vi "WPI_MotorControlOpen NidecBrushless.vi"(6 "Invert":bool, 8 "error in (no error)":errorcluster, 9 "DIO Channel":T1, 10 "PWM Channel":T4) -> (0 "error out":errorcluster, 3 "MotorControlDeviceRef":T2={"DeviceStatus"={"status"=FALSE, "code"=0, "source"=""}, "Type"=enum."PWM", "PWM"={"PWM Channel"=enum."Invalid", "DeadBand"={"Name"="", "maxPositivePwm"=0, "minPositivePwm"=0, "centerPwm"=0, "maxNegativePwm"=0, "minNegativePwm"=0, "angularRange"=0}}, "CAN"={"Device Number"=0, "SetOutput VI Ref"=variant(refnum<vi> refnum), "GetOutput VI Ref"=variant(refnum<vi> refnum), "Enable VI Ref"=variant(refnum<vi> refnum), "Disable VI Ref"=variant(refnum<vi> refnum), "Data"=variant}, "Invert"=FALSE, "DIO PWM"={"PWM \"Enable\" Channel"=enum."Invalid", "DIOChannel"=enum."Invalid", "PWM Rate"=0.0}})   [LabVIEW 2017]
doc: "Creates a reference to the Nidec Brushless motor controller you specify. You must open a reference before using any other VIs on this palette. After you open a reference to the motor controller, you can use the SetOutput and GetOutput VIs to set and get the output voltage of the motor controller, respectively.\n\nThis software is licensed. Open the labview\\readme\\WPI Robotics Library Open Source License.txt file for more information."
uses:
  <vilib>/Rock Robotics/SystemInterfaces/DIO/FPGA_DIOPWMChannel.ctl
  <vilib>/Rock Robotics/WPI/MotorControl/WPI_MotorControlDeviceRef.ctl
  <vilib>/Rock Robotics/WPI/MotorControl/WPI_MotorControlType.ctl
  <vilib>/Rock Robotics/WPI/PWM/WPI_PWMDeadband.ctl
  <vilib>/Rock Robotics/SystemInterfaces/DIO/FPGA_DIOChannel.ctl
  <vilib>/Rock Robotics/SystemInterfaces/NetworkCommunication/NetComm_UsageReport_ResourceType.ctl
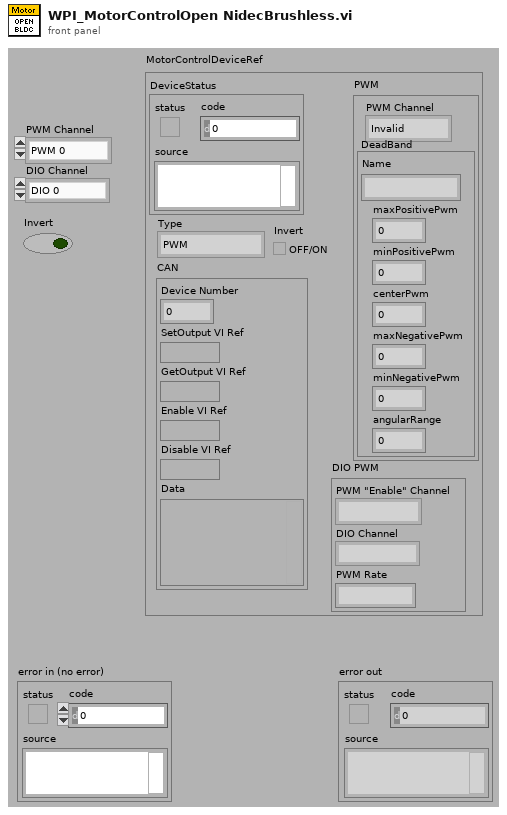
[diagram p1: front panel]
types:
  T1 = typedef "FPGA_DIOChannel.ctl" = enum8{"DIO 0", "DIO 1", "DIO 2", "DIO 3", "DIO 4", "DIO 5", "DIO 6", "DIO 7", "DIO 8", "DIO 9", "DIO MXP 0", "DIO MXP 1", "DIO MXP 2", "DIO MXP 3", "DIO MXP 4", "DIO MXP 5", "DIO MXP 6", "DIO MXP 7", "DIO MXP 8", "DIO MXP 9", "DIO MXP 10", "DIO MXP 11", "DIO MXP 12", "DIO MXP 13", "DIO MXP 14", "DIO MXP 15", "SPI Port CS1", "SPI Port CS2", "SPI Port CS3", "SPI Port MISO", "SPI Port MOSI", "Invalid"}
  T2 = typedef "WPI_MotorControlDeviceRef.ctl" = cluster{"DeviceStatus":errorcluster, "Type":T3, "PWM":cluster{"PWM Channel":T4, "DeadBand":T5}, "CAN":cluster{"Device Number":u8, "SetOutput VI Ref":variant, "GetOutput VI Ref":variant, "Enable VI Ref":variant, "Disable VI Ref":variant, "Data":variant}, "Invert":bool, "DIO PWM":cluster{"PWM \"Enable\" Channel":T4, "DIOChannel":T1, "PWM Rate":dbl}}
  T3 = typedef "WPI_MotorControlType.ctl" = enum16{"PWM", "CAN", "DIO PWM"}
  T4 = typedef "FPGA_DIOPWMChannel.ctl" = enum8{"PWM 0", "PWM 1", "PWM 2", "PWM 3", "PWM 4", "PWM 5", "PWM 6", "PWM 7", "PWM 8", "PWM 9", "PWM MXP 0", "PWM MXP 1", "PWM MXP 2", "PWM MXP 3", "PWM MXP 4", "PWM MXP 5", "PWM MXP 6", "PWM MXP 7", "PWM MXP 8", "PWM MXP 9", "Invalid"}
  T5 = typedef "WPI_PWMDeadband.ctl" = cluster{"Name":string, "maxPositivePwm":i32, "minPositivePwm":i32, "centerPwm":i32, "maxNegativePwm":i32, "minNegativePwm":i32, "angularRange":u16}
  T6 = typedef "NetComm_UsageReport_ResourceType.ctl" = enum8{"Controller", "Module", "Language", "CANPlugin", "Accelerometer", "ADXL345", "AnalogChannel", "AnalogTrigger", "AnalogTriggerOutput", "CANJaguar", "Compressor", "Counter", "Dashboard", "DigitalInput", "DigitalOutput", "DriverStationCIO", "DriverStationEIO", "DriverStationLCD", "Encoder", "GearTooth", "Gyro", "I2C", "Framework", "Jaguar", "Joystick", "Kinect", "KinectStick", "PIDController", "Preferences", "PWM", "Relay", "RobotDrive", "SerialPort", "Servo", "Solenoid", "SPI", "Task", "Ultrasonic", "Victor", "Button", "Command", "AxisCamera", "PCVideoServer", "SmartDashboard", "Talon", "HiTechnicColorSensor", "HiTechnicAccel", "HiTechnicCompass", "SRF08", "AnalogOutput", "Victor SP", "Talon SRX", "CAN Talon SRX", "ADXL362 Accel", "ADXRS450 Gyro", "Rev SPARK", "Mindsensors SD540", "Digital Filter", "ADIS16448", "PDP", "PCM", "PigeonIMU", "Nidec Brushless", "CTRE CANifier", "CTRE Future 0", "CTRE Future 1", "CTRE Future 2", "CTRE Future 3", "CTRE Future 4", "CTRE Future 5", "CTRE Future 6"}
  T7 = typedef "WPI_DigitalOutputDevRef.ctl" = cluster{"DIO Channel":T1, "DevStatus":errorcluster}
  T8 = typedef "WPI_PWMDeviceRef.ctl" = cluster{"DeviceStatus":errorcluster, "PWM Channel":T4}
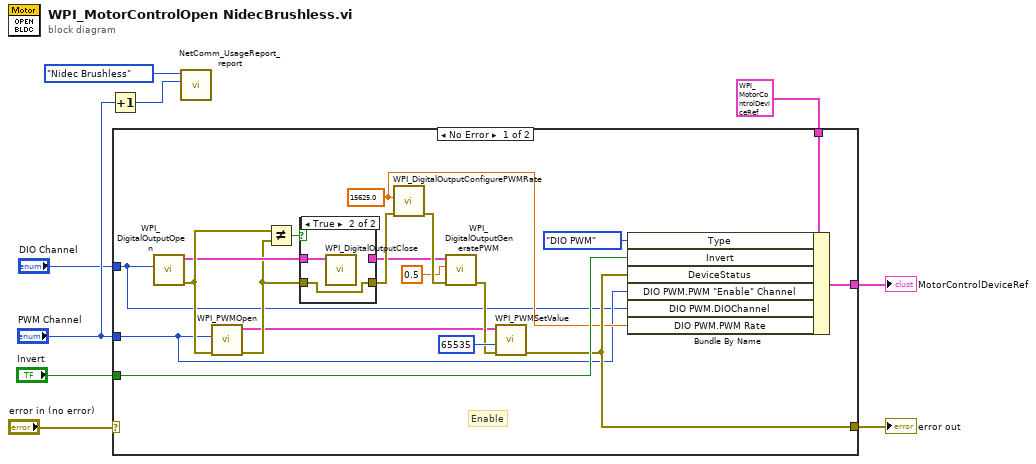
[diagram p0: block diagram]
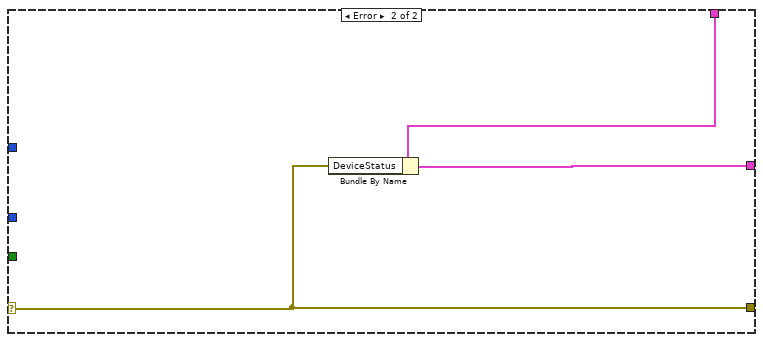
[diagram p3: hidden frame]
diagram:
  n1 = Increment(x="PWM Channel") -> (x+1=w8:T4)
  n2 = case shown="No Error" "error in (no error)" {
    selector: "error in (no error)" -> [_ w33]
    tunnel: "PWM Channel" -> [w11 _]
    tunnel: T2 {"DeviceStatus"={"status"=FALSE, "code"=0, "source"=""}, "Type"=enum."PWM", "PWM"={"PWM Channel"=enum."PWM 0", "DeadBand"={"Name"="", "maxPositivePwm"=0, "minPositivePwm"=0, "centerPwm"=0, "maxNegativePwm"=0, "minNegativePwm"=0, "angularRange"=0}}, "CAN"={"Device Number"=0, "SetOutput VI Ref"=variant(refnum<vi> refnum), "GetOutput VI Ref"=variant(refnum<vi> refnum), "Enable VI Ref"=variant(refnum<vi> refnum), "Disable VI Ref"=variant(refnum<vi> refnum), "Data"=variant}, "Invert"=FALSE, "DIO PWM"={"PWM \"Enable\" Channel"=enum."Invalid", "DIOChannel"=enum."Invalid", "PWM Rate"=0.0}} ("MotorControlDeviceRef") -> [w28 w35]
    tunnel: [w24 w34] -> w5
    tunnel: [w23 w33] -> w4
    tunnel: "Invert" -> [w27 _]
    tunnel: "DIO Channel" -> [w10 _]
    frame No Error {
      w12 = sgl 15625.0 ("PWM Rate (Hz)")
      # "Enable"
      n3 = call <vilib>:"WPI_DigitalOutputOpen.vi"("DIO Channel"=w10) -> ("error out"=w22:errorcluster, "DigitalOutputDevRef"=w20:T7)  [unwired: 9 in]
      n4 = call <vilib>:"WPI_PWMOpen.vi"("error in"=w22, "PWM Channel"=w11) -> ("error out"=w17:errorcluster, "PWMDeviceRef"=w14:T8)  [unwired: 8 in]
      n5 = Not Equal?(x=w22, y=w17) -> (x != y?=w21:bool)
      n6 = case shown="True" w21 {
        tunnel: w20 -> [w30 w32]
        tunnel: w17 -> [w29 w31]
        tunnel: [w30 _] -> w15
        tunnel: [w29 w31] -> w16
        frame False {
        }
        frame True {
          n7 = call <vilib>:"WPI_DigitalOutputClose.vi"("DigitalOutputDevRef"=w32) -> ()  [unwired: 10 in, 1 out]
        }
      }
      n8 = call <vilib>:"WPI_DigitalOutputConfigurePWMRate.vi"("error in (no error)"=w16, "PWM Rate (Hz)"=w12) -> ("error out"=w19:errorcluster)  [unwired: 8 in, 1 out]
      n9 = call <vilib>:"WPI_DigitalOutputGeneratePWM.vi"("error in (no error)"=w19, "PWM Duty Cycle"=sgl 0.5, "DigitalOutputDevRef"=w15) -> ("error out"=w18:errorcluster)  [unwired: 7 in, 1 out]
      n10 = call <vilib>:"WPI_PWMSetValue.vi"("error in (no error)"=w18, "Value"=u16 65535, "PWMDeviceRef"=w14) -> ("error out"=w23:errorcluster)  [unwired: 1 in, 7 out]
      n11 = Bundle By Name(cluster=w28, "Type"=WPI_MotorControlType."DIO PWM", "Invert"=w27, "DeviceStatus"=w23, "DIO PWM.PWM \"Enable\" Channel"=w11, "DIO PWM.DIOChannel"=w10, "DIO PWM.PWM Rate"=w12) -> (w24:T2)
    }
    frame Error {
      n12 = Bundle By Name(cluster=w35, "DeviceStatus"=w33) -> (w34:T2)
    }
  }
  "MotorControlDeviceRef" <- w5
  "error out" <- w4
  n13 = call <vilib>:"NetComm_UsageReport_report.vi"("Instance Number"=w8, "Resource Type"=NetComm_UsageReport_ResourceType."Nidec Brushless") -> ()  [unwired: 10 in]
